vi "BRig_RT__Case_Exp__State_initTrial2__v4.vi"(0 "input_dataCurrent":u16[](array[numeric]), 1 "input_dataTrial":u16[][](array[numeric]), 3 "input_dataExp":u16[](array[numeric]), 6 "input_dataBlock":u16[][](array[numeric]), 8 "input_dataLC":u16[](array[numeric])) -> (7 "output_L_Wrong_Laser_l2":bool, 9 "output_L_Wrong_Event_l2":bool, 10 "output_L_Power_l1":dbl, 11 "output_L_Reward_Laser_l2":bool, 12 "output_L_Power_l2":dbl, 13 "output_L_Reward_Event_l2":bool, 14 "output_dataCurrent":u16[](array[numeric]), 15 "output_dataTrial":u16[][](array[numeric]), 16 "output_L_Reward_Event_l1":bool, 17 "output_L_Reward_Laser_l1":bool, 18 "output_L_Wrong_Event_l1":bool, 19 "output_L_Wrong_Laser_l1":bool)   [LabVIEW 2014]
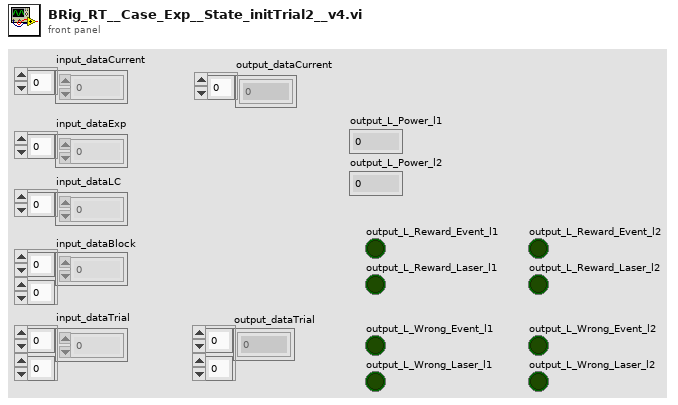
[diagram p1: front panel]
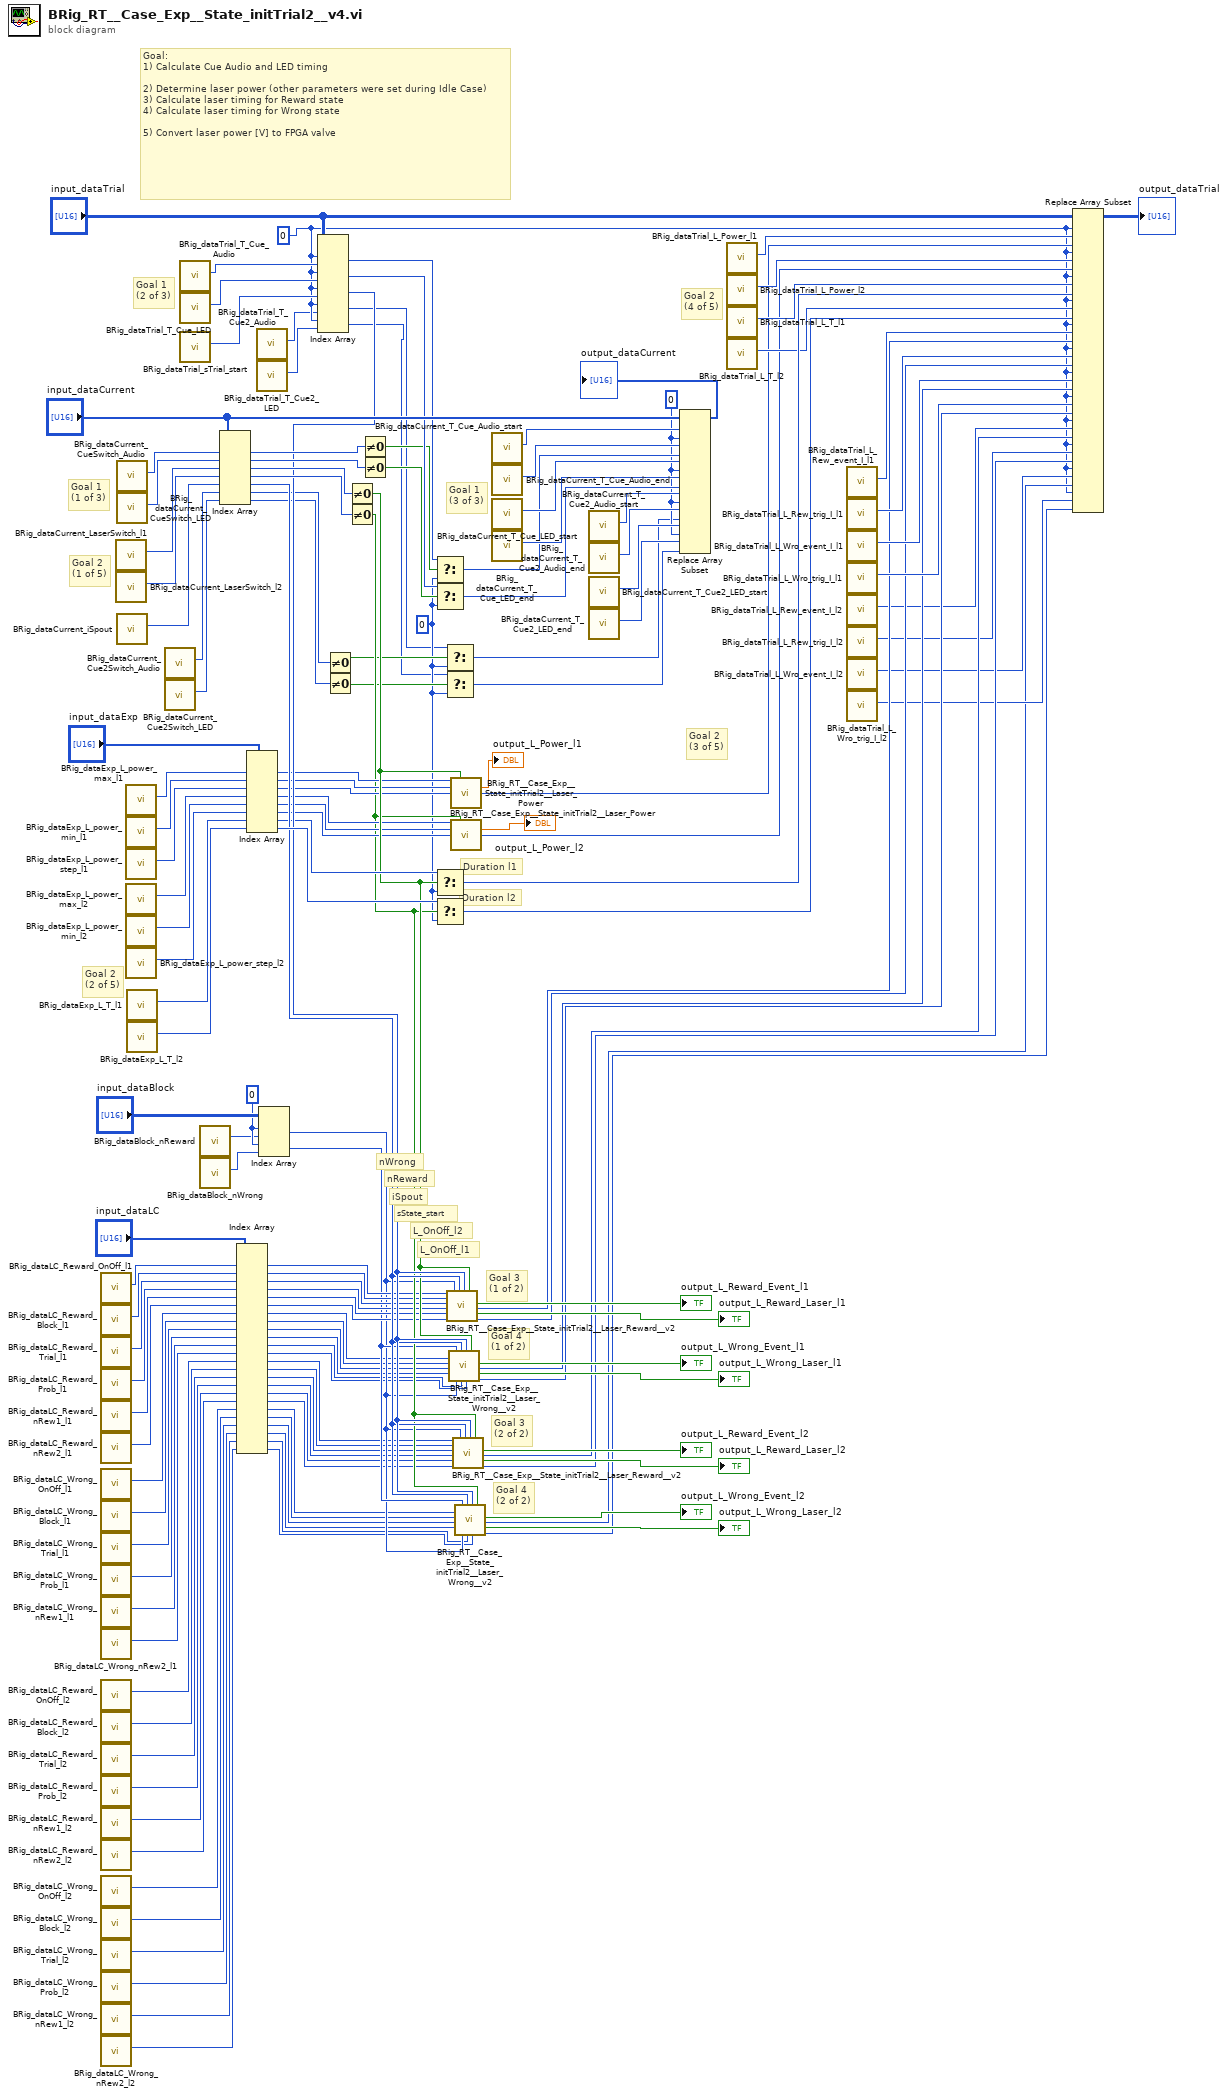
[diagram p0: block diagram]
diagram:
  w48 = 0 ("disabled index (row)")
  w69 = 0
  w60 = u16 0 ("f")
  w53 = u16 0 ("new element/subarray")
  # "nWrong"
  # "nReward"
  # "L_OnOff_l2"
  # "Goal 2\n(3 of 5)"
  # "Goal 4\n(2 of 2)"
  # "Goal 4\n(1 of 2)"
  # "Goal 3\n(2 of 2)"
  # "Goal 3\n(1 of 2)"
  # "L_OnOff_l1"
  # "sState_start"
  # "iSpout"
  # "Goal 2\n(4 of 5)"
  # "Goal 2\n(2 of 5)"
  # "Duration l2"
  # "Duration l1"
  # "Goal 2\n(1 of 5)"
  # "Goal 1\n(3 of 3)"
  # "Goal 1\n(2 of 3)"
  # "Goal 1\n(1 of 3)"
  # "Goal:\n1) Calculate Cue Audio and LED timing\n\n2) Determine laser power (other parameters were set during Idle Case)\n3) Calculate laser timing for Reward state\n4) Calculate laser timing for Wrong state\n\n5) Convert laser power [V] to FPGA valve"
  n1 = call "BRig_dataLC_Reward_OnOff_l1.vi"() -> ("output_Reward_OnOff"=w116:i32)  [unwired: 11 in]
  n2 = call "BRig_dataLC_Reward_Block_l1.vi"() -> ("output_Reward_Block"=w115:i32)  [unwired: 11 in]
  n3 = call "BRig_dataLC_Reward_Trial_l1.vi"() -> ("output_Reward_Trial"=w114:i32)  [unwired: 11 in]
  n4 = call "BRig_dataLC_Reward_Prob_l1.vi"() -> ("output_Reward_Prob"=w113:i32)  [unwired: 11 in]
  n5 = call "BRig_dataLC_Reward_nRew1_l1.vi"() -> ("output_Reward_nRew1_l1"=w42:i32)  [unwired: 11 in]
  n6 = call "BRig_dataLC_Reward_nRew2_l1.vi"() -> ("output_Reward_nRew2_l1"=w41:i32)  [unwired: 11 in]
  n7 = call "BRig_dataLC_Wrong_OnOff_l1.vi"() -> ("output_Wrong_OnOff"=w38:i32)  [unwired: 11 in]
  n8 = call "BRig_dataLC_Wrong_Block_l1.vi"() -> ("output_Wrong_Block"=w37:i32)  [unwired: 11 in]
  n9 = call "BRig_dataLC_Wrong_Trial_l1.vi"() -> ("output_Wrong_Trial"=w36:i32)  [unwired: 11 in]
  n10 = call "BRig_dataLC_Wrong_Prob_l1.vi"() -> ("output_Wrong_Prob"=w35:i32)  [unwired: 11 in]
  n11 = call "BRig_dataLC_Wrong_nRew1_l1.vi"() -> ("output_Wrong_nRew1_l1"=w16:i32)  [unwired: 11 in]
  n12 = call "BRig_dataLC_Wrong_nRew2_l1.vi"() -> ("output_Wrong_nRew2_l1"=w15:i32)  [unwired: 11 in]
  n13 = call "BRig_dataLC_Reward_OnOff_l2.vi"() -> ("output_Reward_OnOff_l2"=w23:i32)  [unwired: 11 in]
  n14 = call "BRig_dataLC_Reward_Block_l2.vi"() -> ("output_Reward_Block_l2"=w24:i32)  [unwired: 11 in]
  n15 = call "BRig_dataLC_Reward_Trial_l2.vi"() -> ("output_Reward_Trial_l2"=w25:i32)  [unwired: 11 in]
  n16 = call "BRig_dataLC_Reward_Prob_l2.vi"() -> ("output_Reward_Prob_l2"=w26:i32)  [unwired: 11 in]
  n17 = call "BRig_dataLC_Reward_nRew1_l2.vi"() -> ("output_Reward_nRew1_l2"=w27:i32)  [unwired: 11 in]
  n18 = call "BRig_dataLC_Reward_nRew2_l2.vi"() -> ("output_Reward_nRew2_l2"=w28:i32)  [unwired: 11 in]
  n19 = call "BRig_dataLC_Wrong_OnOff_l2.vi"() -> ("output_Wrong_OnOff_l2"=w29:i32)  [unwired: 11 in]
  n20 = call "BRig_dataLC_Wrong_Block_l2.vi"() -> ("output_Wrong_Block_l2"=w30:i32)  [unwired: 11 in]
  n21 = call "BRig_dataLC_Wrong_Trial_l2.vi"() -> ("output_Wrong_Trial_l2"=w31:i32)  [unwired: 11 in]
  n22 = call "BRig_dataLC_Wrong_Prob_l2.vi"() -> ("output_Wrong_Prob_l2"=w32:i32)  [unwired: 11 in]
  n23 = call "BRig_dataLC_Wrong_nRew1_l2.vi"() -> ("output_Wrong_nRew1_l2"=w8:i32)  [unwired: 11 in]
  n24 = call "BRig_dataLC_Wrong_nRew2_l2.vi"() -> ("output_Wrong_nRew2_l2"=w7:i32)  [unwired: 11 in]
  n25 = call "BRig_dataCurrent_LaserSwitch_l1.vi"() -> ("output_LaserSwitch_l1"=w140:i32)  [unwired: 11 in]
  n26 = call "BRig_dataCurrent_LaserSwitch_l2.vi"() -> ("output_LaserSwitch_l2"=w139:i32)  [unwired: 11 in]
  n27 = call "BRig_dataCurrent_CueSwitch_Audio.vi"() -> ("output_CueSwitch_Audio"=w155:i32)  [unwired: 11 in]
  n28 = call "BRig_dataCurrent_CueSwitch_LED.vi"() -> ("output_CueSwitch_LED"=w153:i32)  [unwired: 11 in]
  n29 = call "BRig_dataCurrent_iSpout.vi"() -> ("output_iSpout"=w110:i32)  [unwired: 11 in]
  n30 = call "BRig_dataExp_L_power_max_l1.vi"() -> ("output_L_power_max_l1"=w137:i32)  [unwired: 11 in]
  n31 = call "BRig_dataExp_L_power_min_l1.vi"() -> ("output_L_power_min_l1"=w136:i32)  [unwired: 11 in]
  n32 = call "BRig_dataExp_L_power_step_l1.vi"() -> ("output_L_power_step_l1"=w135:i32)  [unwired: 11 in]
  n33 = call "BRig_dataExp_L_power_max_l2.vi"() -> ("output_L_power_max_l2"=w134:i32)  [unwired: 11 in]
  n34 = call "BRig_dataExp_L_power_min_l2.vi"() -> ("output_L_power_min_l2"=w133:i32)  [unwired: 11 in]
  n35 = call "BRig_dataExp_L_power_step_l2.vi"() -> ("output_L_power_step_l2"=w132:i32)  [unwired: 11 in]
  n36 = call "BRig_dataExp_L_T_l1.vi"() -> ("output_L_T_l1"=w131:i32)  [unwired: 11 in]
  n37 = call "BRig_dataExp_L_T_l2.vi"() -> ("output_L_T_l2"=w130:i32)  [unwired: 11 in]
  n38 = call "BRig_dataCurrent_Cue2Switch_Audio.vi"() -> ("output_Cue2Switch_Audio"=w66:i32)  [unwired: 11 in]
  n39 = call "BRig_dataCurrent_Cue2Switch_LED.vi"() -> ("output_Cue2Switch_LED"=w65:i32)  [unwired: 11 in]
  n40 = call "BRig_dataTrial_T_Cue_Audio.vi"() -> ("output_T_Cue_Audio"=w145:i32)  [unwired: 11 in]
  n41 = call "BRig_dataTrial_T_Cue_LED.vi"() -> ("output_T_Cue_LED"=w144:i32)  [unwired: 11 in]
  n42 = call "BRig_dataTrial_sTrial_start.vi"() -> ("output_sTrial_start"=w109:i32)  [unwired: 11 in]
  n43 = call "BRig_dataBlock_nReward.vi"() -> ("output_nReward"=w47:i32)  [unwired: 11 in]
  n44 = call "BRig_dataBlock_nWrong.vi"() -> ("output_nWrong"=w49:i32)  [unwired: 11 in]
  n45 = Index Array(array="input_dataCurrent", index #1=w155, index #2=w153, index #3=w140, index #4=w139, index #5=w110, index #6=w66, index #7=w65) -> (element #1=w148:u16, element #2=w147:u16, element #3=w112:u16, element #4=w111:u16, element #5=w107:u16, element #6=w64:u16, element #7=w63:u16)
  n46 = Index Array(array="input_dataLC", index #1=w116, index #2=w115, index #3=w114, index #4=w113, index #5=w42, index #6=w41, index #7=w38, index #8=w37, index #9=w36, index #10=w35, index #11=w16, index #12=w15, index #13=w23, index #14=w24, index #15=w25, index #16=w26, index #17=w27, index #18=w28, index #19=w29, index #20=w30, index #21=w31, index #22=w32, index #23=w8, index #24=w7) -> (element #1=w46:u16, element #2=w45:u16, element #3=w44:u16, element #4=w43:u16, element #5=w40:u16, element #6=w39:u16, element #7=w14:u16, element #8=w13:u16, element #9=w12:u16, element #10=w11:u16, element #11=w10:u16, element #12=w9:u16, element #13=w17:u16, element #14=w18:u16, element #15=w19:u16, element #16=w20:u16, element #17=w21:u16, element #18=w22:u16, element #19=w6:u16, element #20=w5:u16, element #21=w4:u16, element #22=w3:u16, element #23=w2:u16, element #24=w1:u16)
  n47 = Index Array(array="input_dataExp", index #1=w137, index #2=w136, index #3=w135, index #4=w134, index #5=w133, index #6=w132, index #7=w131, index #8=w130) -> (element #1=w80:u16, element #2=w79:u16, element #3=w78:u16, element #4=w75:u16, element #5=w74:u16, element #6=w73:u16, element #7=w82:u16, element #8=w127:u16)
  n48 = call "BRig_dataTrial_T_Cue2_Audio.vi"() -> ("output_T_Cue2_Audio"=w68:i32)  [unwired: 11 in]
  n49 = call "BRig_dataTrial_T_Cue2_LED.vi"() -> ("output_T_Cue2_LED"=w67:i32)  [unwired: 11 in]
  n50 = Index Array(array="input_dataBlock", index (row) #1=w48, index (col) #1=w47, index (row) #2=w48, index (col) #2=w49) -> (element #1=w33:u16, element #2=w34:u16)
  n51 = Index Array(array="input_dataTrial", index (row) #1=w69, index (col) #1=w145, index (row) #2=w69, index (col) #2=w144, index (row) #3=w69, index (col) #3=w109, index (row) #4=w69, index (col) #4=w68, index (row) #5=w69, index (col) #5=w67) -> (element #1=w143:u16, element #2=w142:u16, element #3=w108:u16, element #4=w59:u16, element #5=w58:u16)
  n52 = Not Equal To 0?(x=w64) -> (x != 0?=w62:bool)
  n53 = Not Equal To 0?(x=w63) -> (x != 0?=w61:bool)
  n54 = Not Equal To 0?(x=w112) -> (x != 0?=w81:bool)
  n55 = Not Equal To 0?(x=w111) -> (x != 0?=w72:bool)
  n56 = Not Equal To 0?(x=w148) -> (x != 0?=w129:bool)
  n57 = Not Equal To 0?(x=w147) -> (x != 0?=w128:bool)
  n58 = Select(t=w143, s=w129, f=w60) -> (s? t:f=w146:u16)
  n59 = Select(t=w142, s=w128, f=w60) -> (s? t:f=w141:u16)
  n60 = Select(t=w82, s=w81, f=w60) -> (s? t:f=w120:u16)
  n61 = Select(t=w127, s=w72, f=w60) -> (s? t:f=w118:u16)
  n62 = Select(t=w59, s=w62, f=w60) -> (s? t:f=w52:u16)
  n63 = Select(t=w58, s=w61, f=w60) -> (s? t:f=w51:u16)
  n64 = call "BRig_RT__Case_Exp__State_initTrial2__Laser_Reward__v2.vi"("input_L_OnOff"=w46, "input_L_Block"=w45, "input_L_Trial"=w44, "input_L_Probability"=w43, "input_L_nRew1"=w40, "input_L_nRew2"=w39, "input_nReward"=w33, "input_iSpout"=w107, "input_sState_start"=w108, "input_LaserSwitch"=w81) -> ("output_LR_Event"=→"output_L_Reward_Event_l1":bool, "output_LR_Event_num"=w94:u16, "output_LR_Laser"=→"output_L_Reward_Laser_l1":bool, "output_LR_Laser_num"=w93:u16)  [unwired: 6 in]
  n65 = call "BRig_RT__Case_Exp__State_initTrial2__Laser_Wrong__v2.vi"("input_L_OnOff"=w14, "input_L_Block"=w13, "input_L_Trial"=w12, "input_L_Probability"=w11, "input_nWrong"=w34, "input_nReward"=w33, "input_iSpout"=w107, "input_L_nRew1"=w10, "input_sState_start"=w108, "input_L_nRew2"=w9, "input_LaserSwitch"=w81) -> ("output_LR_Event"=→"output_L_Wrong_Event_l1":bool, "output_LR_Event_num"=w92:u16, "output_LR_Laser"=→"output_L_Wrong_Laser_l1":bool, "output_LR_Laser_num"=w91:u16)  [unwired: 5 in]
  n66 = call "BRig_RT__Case_Exp__State_initTrial2__Laser_Power.vi"("input_L_Power_max__x100"=w80, "input_LaserSwitch"=w81, "input_L_Power_min__x100"=w79, "input_L_Power_step__x100"=w78) -> ("output_L_Power"=→"output_L_Power_l1":dbl, "output_L_Power_x100"=w76:u16)  [unwired: 10 in]
  n67 = call "BRig_RT__Case_Exp__State_initTrial2__Laser_Power.vi"("input_L_Power_max__x100"=w75, "input_LaserSwitch"=w72, "input_L_Power_min__x100"=w74, "input_L_Power_step__x100"=w73) -> ("output_L_Power"=→"output_L_Power_l2":dbl, "output_L_Power_x100"=w70:u16)  [unwired: 10 in]
  n68 = call "BRig_RT__Case_Exp__State_initTrial2__Laser_Reward__v2.vi"("input_L_OnOff"=w17, "input_L_Block"=w18, "input_L_Trial"=w19, "input_L_Probability"=w20, "input_L_nRew1"=w21, "input_L_nRew2"=w22, "input_nReward"=w33, "input_iSpout"=w107, "input_sState_start"=w108, "input_LaserSwitch"=w72) -> ("output_LR_Event"=→"output_L_Reward_Event_l2":bool, "output_LR_Event_num"=w89:u16, "output_LR_Laser"=→"output_L_Reward_Laser_l2":bool, "output_LR_Laser_num"=w87:u16)  [unwired: 6 in]
  n69 = call "BRig_RT__Case_Exp__State_initTrial2__Laser_Wrong__v2.vi"("input_L_OnOff"=w6, "input_L_Block"=w5, "input_L_Trial"=w4, "input_L_Probability"=w3, "input_nWrong"=w34, "input_nReward"=w33, "input_iSpout"=w107, "input_L_nRew1"=w2, "input_sState_start"=w108, "input_L_nRew2"=w1, "input_LaserSwitch"=w72) -> ("output_LR_Event"=→"output_L_Wrong_Event_l2":bool, "output_LR_Event_num"=w84:u16, "output_LR_Laser"=→"output_L_Wrong_Laser_l2":bool, "output_LR_Laser_num"=w83:u16)  [unwired: 5 in]
  n70 = call "BRig_dataCurrent_T_Cue_Audio_start.vi"() -> ("output_T_Cue_Audio_start"=w152:i32)  [unwired: 11 in]
  n71 = call "BRig_dataCurrent_T_Cue_Audio_end.vi"() -> ("output_T_Cue_Audio_end"=w151:i32)  [unwired: 11 in]
  n72 = call "BRig_dataCurrent_T_Cue_LED_start.vi"() -> ("output_T_Cue_LED_start"=w150:i32)  [unwired: 11 in]
  n73 = call "BRig_dataCurrent_T_Cue_LED_end.vi"() -> ("output_T_Cue_LED_end"=w149:i32)  [unwired: 11 in]
  n74 = call "BRig_dataCurrent_T_Cue2_Audio_start.vi"() -> ("output_T_Cue2_Audio_start"=w57:i32)  [unwired: 11 in]
  n75 = call "BRig_dataCurrent_T_Cue2_Audio_end.vi"() -> ("output_T_Cue2_Audio_end"=w56:i32)  [unwired: 11 in]
  n76 = call "BRig_dataCurrent_T_Cue2_LED_start.vi"() -> ("output_T_Cue2_LED_start"=w55:i32)  [unwired: 11 in]
  n77 = call "BRig_dataCurrent_T_Cue2_LED_end.vi"() -> ("output_T_Cue2_LED_end"=w54:i32)  [unwired: 11 in]
  n78 = Replace Array Subset(array="input_dataCurrent", new element #1=w53, index #1=w152, new element #2=w146, index #2=w151, new element #3=w53, index #3=w150, new element #4=w141, index #4=w149, new element #5=w53, index #5=w57, new element #6=w52, index #6=w56, new element #7=w53, index #7=w55, new element #8=w51, index #8=w54) -> (→"output_dataCurrent":u16[])
  n79 = call "BRig_dataTrial_L_Power_l1.vi"() -> ("output_L_Power_l1"=w123:i32)  [unwired: 11 in]
  n80 = call "BRig_dataTrial_L_Power_l2.vi"() -> ("output_L_Power_l2"=w122:i32)  [unwired: 11 in]
  n81 = call "BRig_dataTrial_L_T_l1.vi"() -> ("output_L_T_l1"=w121:i32)  [unwired: 11 in]
  n82 = call "BRig_dataTrial_L_T_l2.vi"() -> ("output_L_T_l2"=w119:i32)  [unwired: 11 in]
  n83 = call "BRig_dataTrial_L_Rew_event_I_l1.vi"() -> ("output_L_Rew_event_I_l1"=w102:i32)  [unwired: 11 in]
  n84 = call "BRig_dataTrial_L_Rew_trig_I_l1.vi"() -> ("output_L_Rew_trig_I_l1"=w101:i32)  [unwired: 11 in]
  n85 = call "BRig_dataTrial_L_Wro_event_I_l1.vi"() -> ("output_L_Wro_event_I_l1"=w100:i32)  [unwired: 11 in]
  n86 = call "BRig_dataTrial_L_Wro_trig_I_l1.vi"() -> ("output_L_Wro_trig_I_l1"=w99:i32)  [unwired: 11 in]
  n87 = call "BRig_dataTrial_L_Rew_event_I_l2.vi"() -> ("output_L_Rew_event_I_l2"=w90:i32)  [unwired: 11 in]
  n88 = call "BRig_dataTrial_L_Rew_trig_I_l2.vi"() -> ("output_L_Rew_trig_I_l2"=w88:i32)  [unwired: 11 in]
  n89 = call "BRig_dataTrial_L_Wro_event_I_l2.vi"() -> ("output_L_Wro_event_I_l2"=w86:i32)  [unwired: 11 in]
  n90 = call "BRig_dataTrial_L_Wro_trig_I_l2.vi"() -> ("output_L_Wro_trig_I_l2"=w85:i32)  [unwired: 11 in]
  n91 = Replace Array Subset(array="input_dataTrial", new element #1=w76, index (row) #1=w69, index (col) #1=w123, new element #2=w70, index (row) #2=w69, index (col) #2=w122, new element #3=w120, index (row) #3=w69, index (col) #3=w121, new element #4=w118, index (row) #4=w69, index (col) #4=w119, new element #5=w94, index (row) #5=w69, index (col) #5=w102, new element #6=w93, index (row) #6=w69, index (col) #6=w101, new element #7=w92, index (row) #7=w69, index (col) #7=w100, new element #8=w91, index (row) #8=w69, index (col) #8=w99, new element #9=w89, index (row) #9=w69, index (col) #9=w90, new element #10=w87, index (row) #10=w69, index (col) #10=w88, new element #11=w84, index (row) #11=w69, index (col) #11=w86, new element #12=w83, index (row) #12=w69, index (col) #12=w85) -> (→"output_dataTrial":u16[][])
